vi "GE 5565PIORC.Registers.LCSR1.Window 1.Get.vi"(8 "error in (no error)":errorcluster, 11 "GE 5565PIORC in":refnum<class "GE 5565PIORC.lvclass">) -> (0 "error out":errorcluster, 2 "Window 1":bool, 3 "GE 5565PIORC out":refnum<class "GE 5565PIORC.lvclass">)   [LabVIEW 2016, in "GE 5565PIORC.lvclass"]
doc: "The PCI PIO window size is selected by setting S1 switch positions 3 and 4. Bit 19 (Window 0) is connected to S1 switch position 3 (‘1’ when ON, ‘0’ when OFF). Bit 22 (Window 1) is connected to S1 switch position 4 (‘1’ when ON, ‘0’ when OFF). These two bits indicate the memory PCI PIO window size as defined in the following table. The two bits are read only.\n\n<B>Bits</B> <B>Window Size</B>\n00 Default = installed memory size\n01 64 MB\n10 16 MB\n11 2 MB"
uses:
  GE 5565PIORC.lvclass
  GE 5565PIORC.Registers.RFM Control and Status.ctl
  GE 5565PIORC.lvclass/GE 5565PIORC.ctl
  GE 5565PIORC.Register.RFM Control and Status.Read (U32).vi
  GE 5565PIORC.Register.Read.vi
  GE 5565PIORC.Register.Read (U32).vi
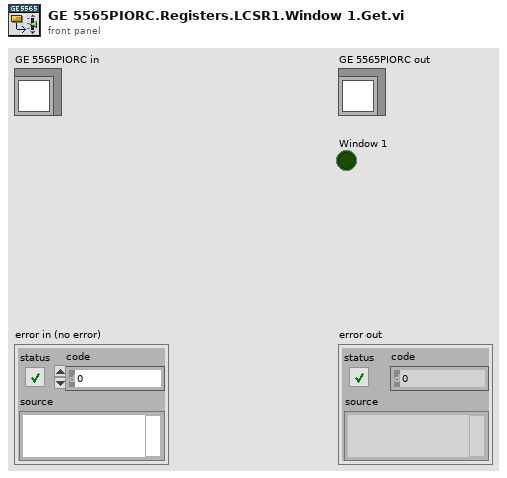
[diagram p1: front panel]
types:
  T1 = typedef "GE 5565PIORC.lvclass/GE 5565PIORC.Registers.RFM Control and Status.ctl" = u32
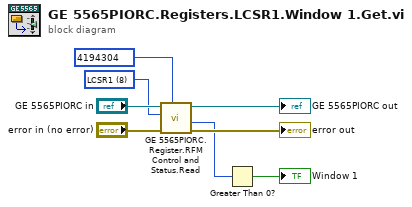
[diagram p0: block diagram]
diagram:
  w4 = T1 8 items=["BRV"=0, "BID"=1, "BRB"=2, "NID"=4, "LCSR1"=8, "LISR"=16, "LIER"=20, "NTD"=24, "NTN"=28, "NIC"=29, "ISD1"=32, "SID1"=36, "ISD2"=40, "SID2"=44, "ISD3"=48, "SID3"=52, "ISD4"=56, "SID4"=60] ("Register")
  n1 = call-poly "GE 5565PIORC.Register.RFM Control and Status.Read.vi"("Mask (0xFFFFFFFF)"=u32 4194304, "error in (no error)"="error in (no error)", "Register"=w4, "GE 5565PIORC in"="GE 5565PIORC in") -> ("error out"=→"error out":errorcluster, "Value"=w1:u32, "GE 5565PIORC out"=→"GE 5565PIORC out":refnum<class "GE 5565PIORC.lvclass">)  [unwired: 5 in]
  n2 = Greater Than 0?(x=w1) -> (x > 0?=→"Window 1":bool)
